vi "Make Element Blink.vi"(8 "error in (no error)":errorcluster, 9 "Colour":u32(colorbox), 10 "Board Game in":refnum<class "Board Game.lvclass">, 11 "GameEl in":refnum<class "GameEl.lvclass">) -> (0 "error out":errorcluster, 1 "Blink Values":u32[][](array[numeric]), 2 "Current Values":u32[][](array[numeric]), 3 "GameEl out":refnum<class "GameEl.lvclass">)   [LabVIEW 2021, in "GameEl.lvclass"]
uses:
  GameEl.lvclass
  Board Game_class/Board Game.lvclass
  GameEl.lvclass/GameEl.ctl
  Board Game_class/Board Game.lvclass/Board Game.ctl
  Board Game_class/Read Board Game Vals.vi
  Board Game_class/Read Board Game Ref.vi
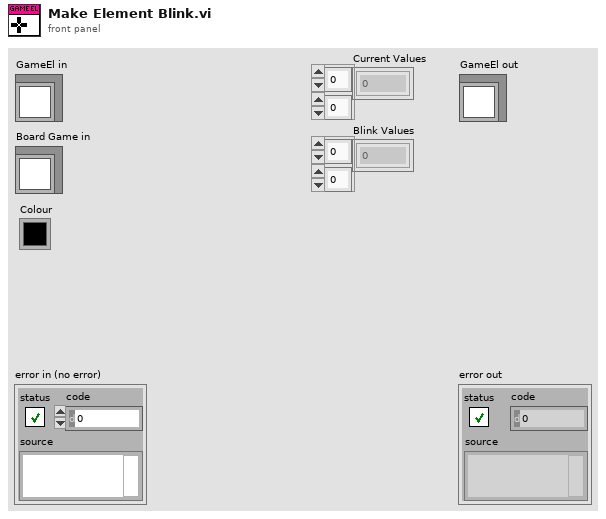
[diagram p1: front panel]
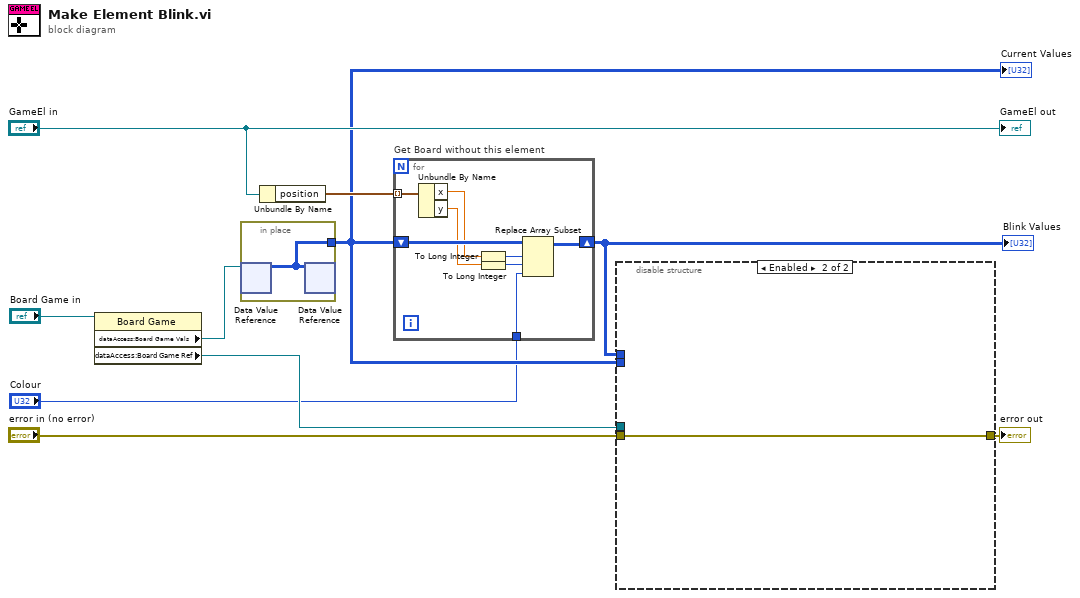
[diagram p0: block diagram]
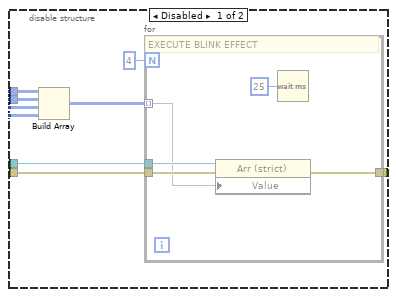
[diagram p2: hidden frame]
diagram:
  n1 = property class="Board Game"(reference="Board Game in") -> ("dataAccess:Board Game Vals"=w4:refnum<data-value>, "dataAccess:Board Game Ref"=w2:refnum<vi>)  [unwired: 1 in, 2 out]
  n2 = in-place {
    in-place-border: [w11] -> w3
    n3 = in-place-dvr #1(w4) -> (w11:u32[][])  [unwired: 1 out]
    n4 = in-place-dvr #1(w11) -> ()  [unwired: 2 out]
  }
  "Current Values" <- w3
  n5 = Unbundle By Name("GameEl in") -> ("position"=w9:cluster{"x":dbl, "y":dbl}[])
  n6 = for "Get Board without this element" {
    tunnel: w9 -> [w17] mode=indexing
    shift-right: [w18] -> w6
    shift-left: w3 -> [w19]
    tunnel: "Colour" -> [w12]
    n7 = Unbundle By Name(w17) -> ("x"=w16:dbl, "y"=w15:dbl)
    n8 = To Long Integer(number=w16) -> (32bit integer=w14:i32)
    n9 = To Long Integer(number=w15) -> (32bit integer=w13:i32)
    n10 = Replace Array Subset(array=w19, new element=w12, index (row)=w14, index (col)=w13) -> (w18:u32[][])
  }
  "Blink Values" <- w6
  n11 = disable-structure shown="Enabled" {
    disable-tunnel: "error in (no error)" -> [w26 w32]
    disable-tunnel: [w25 w32] -> w7
    disable-tunnel: w6 -> [w23 _]
    disable-tunnel: w2 -> [w21 _]
    disable-tunnel: w3 -> [w20 _]
    frame Disabled {
      n12 = Build Array(w23, w20, w23, w20) -> (w22:u32[][][])
      n13 = for {
        N: 4 -> [_]
        tunnel: w26 -> [w31]
        tunnel: [w30] -> w25
        tunnel: w22 -> [w28] mode=indexing
        tunnel: w21 -> [w29]
        # "EXECUTE BLINK EFFECT"
        n14 = property class="Arr (strict)"(reference=w29, error in=w31, "Value"=w28) -> (error out=w30:errorcluster)  [unwired: 1 out]
        n15 = Wait (ms)(milliseconds to wait=u32 25) -> ()  [unwired: 1 out]
      }
    }
    frame Enabled {
    }
  }
  "error out" <- w7
  "GameEl out" <- "GameEl in"
